vi "Return Events.vi"(8 "error in (no error)":errorcluster, 10 "Event Reply Queue":refnum<queue>, 11 "Command Handler in":refnum<class "Command Handler.lvclass">) -> (0 "error out":errorcluster, 3 "Command Handler out":refnum<class "Command Handler.lvclass">)   [LabVIEW 2017, in "Command Handler.lvlib" / "Command Handler.lvclass"]
uses:
  Command Handler.lvclass
  Type Defs/Event Cluster.ctl
  Command Parents/Command.lvclass
  Type Defs/Command Handler Data.ctl
  Command Handler.lvclass/Command Handler.ctl
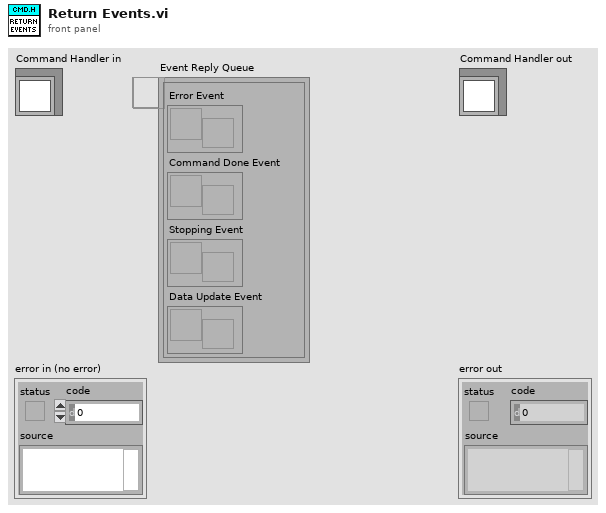
[diagram p1: front panel]
types:
  T1 = typedef "Command Handler.lvlib/Command Handler.lvclass/Event Cluster.ctl" = cluster{"Error Event":refnum<user-event>, "Command Done Event":refnum<user-event>, "Stopping Event":refnum<user-event>, "Data Update Event":refnum<user-event>}
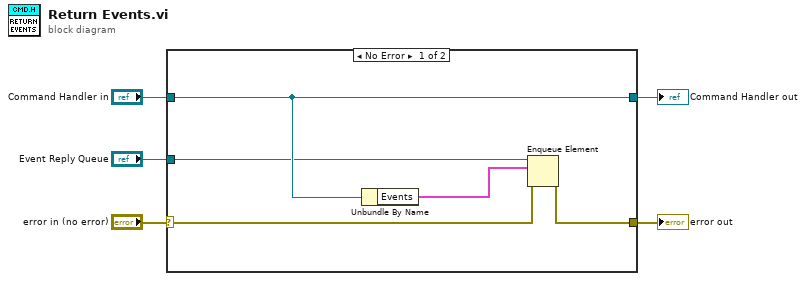
[diagram p0: block diagram]
diagram:
  n1 = case shown="No Error" "error in (no error)" {
    selector: "error in (no error)" -> [w10 w12]
    tunnel: [w9 w12] -> w4
    tunnel: [w8 w11] -> w2
    tunnel: "Command Handler in" -> [w8 w11]
    tunnel: "Event Reply Queue" -> [w6 _]
    frame No Error {
      n2 = Unbundle By Name(w8) -> ("Events"=w7:T1)
      n3 = Enqueue Element(queue=w6, element=w7, error in (no error)=w10) -> (error out=w9:errorcluster)  [unwired: 1 in, 2 out]
    }
    frame Error {
    }
  }
  "error out" <- w4
  "Command Handler out" <- w2
